vi "MenuItemConstructor.vi"   [LabVIEW 2016, in "MGI_MenuItem.lvclass"]
doc: "Use this to create a new MenuItem. Most of the menu items you create can be left as generic menu items. Only use a specialized menu item when you need to use an additional field of that menu item. For example a shortcut in a VI MenuItem, or an icon in a MenuStrip MenuItem\n\nAuthored by Derek E. Trepanier\nsupport@mooregoodideas.com\nwww.mooregoodideas.com\n\nCopyright (c) 2012, Moore Good Ideas, Inc.\n\nAll rights reserved.\n\nRedistribution and use in source and binary forms, with or without modification, are permitted provided that the following conditions are met:\n\n * Redistributions of source code must retain the above copyright notice, this list of conditions and the following disclaimer.\n * Redistributions in binary form must reproduce the above copyright notice, this list of conditions and the following disclaimer in the documentation and/or other materials provided with the distribution.\n * Neither the name of Moore Good Ideas, Inc. nor the names of its contributors may be used to endorse or promote products derived from this software without specific prior written permission.\n\nTHIS SOFTWARE IS PROVIDED BY THE COPYRIGHT HOLDERS AND CONTRIBUTORS \"AS IS\" AND ANY EXPRESS OR IMPLIED WARRANTIES, INCLUDING, BUT NOT LIMITED TO, THE IMPLIED WARRANTIES OF MERCHANTABILITY AND FITNESS FOR A PARTICULAR PURPOSE ARE DISCLAIMED. IN NO EVENT SHALL THE COPYRIGHT OWNER OR CONTRIBUTORS BE LIABLE FOR ANY DIRECT, INDIRECT, INCIDENTAL, SPECIAL, EXEMPLARY, OR CONSEQUENTIAL DAMAGES (INCLUDING, BUT NOT LIMITED TO, PROCUREMENT OF SUBSTITUTE GOODS OR SERVICES; LOSS OF USE, DATA, OR PROFITS; OR BUSINESS INTERRUPTION) HOWEVER CAUSED AND ON ANY THEORY OF LIABILITY, WHETHER IN CONTRACT, STRICT LIABILITY, OR TORT (INCLUDING NEGLIGENCE OR OTHERWISE) ARISING IN ANY WAY OUT OF THE USE OF THIS SOFTWARE, EVEN IF ADVISED OF THE POSSIBILITY OF SUCH DAMAGE."
uses:
  <userlib>/_MGI/Menu Building/MenuItem/MGI_MenuItem.lvclass
  <userlib>/_MGI/Menu Building/MenuItem/VIItem/MGI_VIItem.lvclass
  <userlib>/_MGI/Menu Building/MenuItem/MenuSeparatorItem/MGI_MenuSeparatorItem.lvclass
  <userlib>/_MGI/Menu Building/MenuItem/TrayIcon/MGI_TrayItem.lvclass
  <userlib>/_MGI/Menu Building/MenuItem/MenuStripItem/MGI_MenuStripItem.lvclass
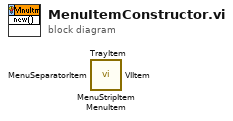
[diagram p0: block diagram]
diagram:
  n1 = call <userlib>:"MenuStripItem.vi"() -> ()  [unwired: 10 in, 2 out]
  n2 = call <userlib>:"TrayItem.vi"() -> ()  [unwired: 10 in, 2 out]
  n3 = call <userlib>:"MenuSeparatorItem.vi"() -> ()  [unwired: 10 in, 2 out]
  n4 = call <userlib>:"VIItem.vi"() -> ()  [unwired: 10 in, 2 out]
  n5 = call <userlib>:"MenuItem.vi"() -> ()  [unwired: 10 in, 2 out]
